vi "SSHDialog.vi"(11 "Slide":u8(slide) scale=0.0..100.0) -> ()   [LabVIEW 2019]
panel:
  # "connected"
  # "start \nmicropython"
  # "Init"
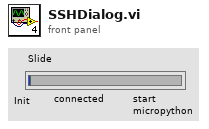
[diagram p1: front panel]
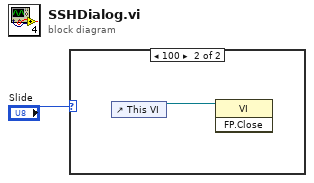
[diagram p0: block diagram]
diagram:
  n1 = case shown="100" "Slide" {
    frame 0, Default {
    }
    frame 100 {
      n2 = control-ref of="This VI"() -> (w2:refnum<vi>)
      n3 = invoke class="VI" method="FP.Close"(reference=w2) -> ()  [unwired: 2 in, 3 out]
    }
  }
